vi "write.vi"(9 "Tiempo de Muestreo":string(combo), 10 "Jump Button 3":bool, 11 "Jump Button 4":bool) -> (3 "String":string)   [LabVIEW 2017]
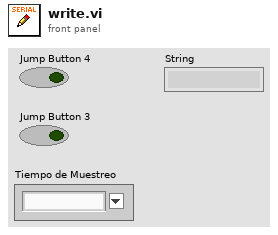
[diagram p1: front panel]
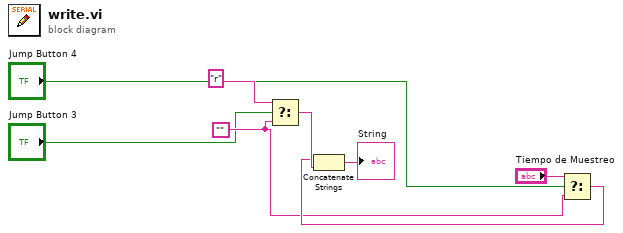
[diagram p0: block diagram]
diagram:
  w2 = ""
  n1 = Select(t="r", s="Jump Button 3", f=w2) -> (s? t:f=w5:string)
  n2 = Select(t="Tiempo de Muestreo", s="Jump Button 4", f=w2) -> (s? t:f=w4:string)
  n3 = Concatenate Strings(w4, w5) -> (→"String":string)
